vi "Create All Message Queues.vi"(8 "error in (no error)":errorcluster, 11 "Process Name":string) -> (0 "error out":errorcluster, 3 "Message Queues":T1)   [LabVIEW 2018, in "4-20mA Module.lvlib"]
uses:
  4-20mA Module.lvlib
  Controls/4-20mA Message Queues.ctl
  support/Message Queue/Message Cluster.ctl
  Config Module/Controls/OP Window Display.ctl
  Controls/4-20mA Display Cluster.ctl
  support/Message Queue/Enqueue Message (Single).vi
  support/Message Queue/Message Queue.lvlib
  Feed Module/Feed Module.lvlib
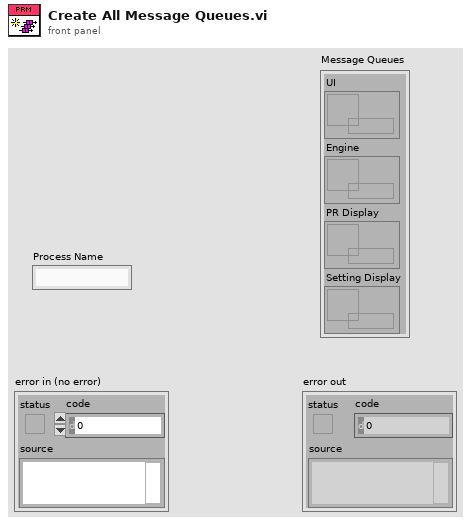
[diagram p1: front panel]
types:
  T1 = typedef "4-20mA Module.lvlib/4-20mA Message Queues.ctl" = cluster{"UI":refnum<queue>, "Engine":refnum<queue>, "PR Display":refnum<queue>, "Setting Display":refnum<queue>}
  T2 = typedef "4-20mA Module.lvlib/4-20mA Display Cluster.ctl" = cluster{"Input 4-20":dbl, "Output 4-20":dbl, "Cycle Period":dbl, "Status":enum16{"Off", "On", "Not Initialized"}}
  T3 = typedef "Feed Module.lvlib/OP Window Display.ctl" = cluster{"Flow":dbl, "Manual":dbl, "Pump Status":u16}
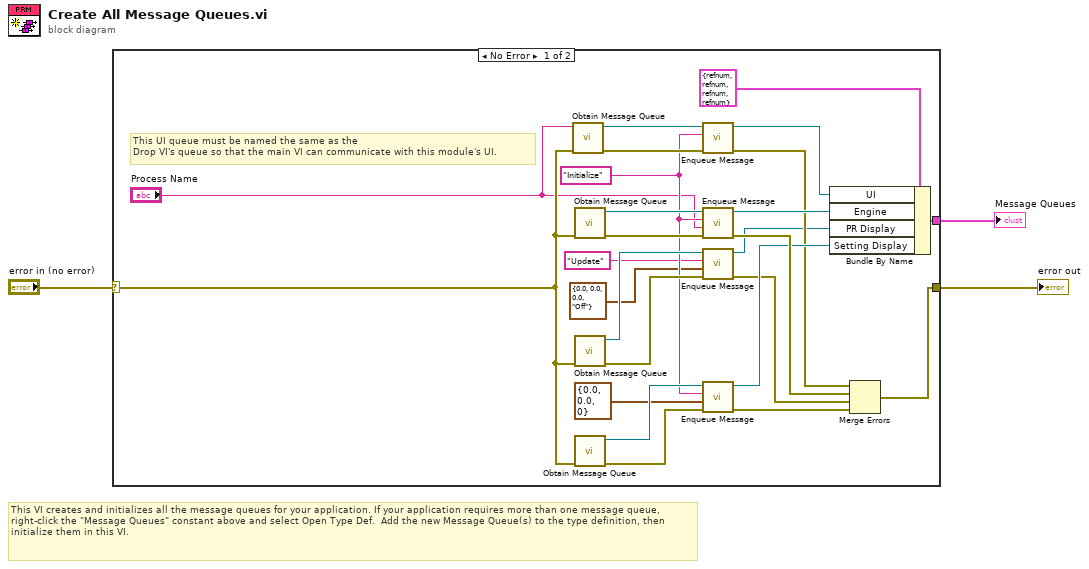
[diagram p0: block diagram]
diagram:
  # "This VI creates and initializes all the message queues for your application. If your application requires more than one message queue, right-click the \"Message Queues\" constant above and select Open Type Def.  Add the new Message Queue(s) to the type definition, then initialize them in this VI."
  n1 = case shown="No Error" "error in (no error)" {
    selector: "error in (no error)" -> [w14 w29]
    tunnel: [w25 w29] -> w3
    tunnel: [w28 _] -> w2
    frame No Error {
      w11 = "Initialize" ("Message")
      # "This UI queue must be named the same as the \nDrop VI's queue so that the main VI can communicate with this module's UI."
      n2 = call "Obtain Message Queue.vi"("error in (no error)"=w14, "name (unnamed)"="Process Name") -> ("error out"=w27:errorcluster, "Message Queue"=w26:refnum<queue>)  [unwired: 8 in]
      n3 = call "Obtain Message Queue.vi"("error in (no error)"=w14) -> ("error out"=w23:errorcluster, "Message Queue"=w24:refnum<queue>)  [unwired: 9 in]
      n4 = call "Obtain Message Queue.vi"("error in (no error)"=w14) -> ("error out"=w20:errorcluster, "Message Queue"=w19:refnum<queue>)  [unwired: 9 in]
      n5 = call "Obtain Message Queue.vi"("error in (no error)"=w14) -> ("error out"=w18:errorcluster, "Message Queue"=w17:refnum<queue>)  [unwired: 9 in]
      n6 = call-poly "Enqueue Message.vi"("error in (no error)"=w27, "Message"=w11, "Message Queue"=w26) -> ("error out"=w8:errorcluster, "dup Message Queue"=w9:refnum<queue>)  [unwired: 7 in]
      n7 = call-poly "Enqueue Message.vi"("error in (no error)"=w23, "Message Data"="Process Name", "Message"=w11, "Message Queue"=w24) -> ("error out"=w21:errorcluster, "dup Message Queue"=w22:refnum<queue>)  [unwired: 6 in]
      n8 = call-poly "Enqueue Message.vi"("error in (no error)"=w20, "Message Data"=T2 {"Input 4-20"=0.0, "Output 4-20"=0.0, "Cycle Period"=0.0, "Status"=enum."Off"} ("PRM Display Cluster"), "Message"="Update", "Message Queue"=w19) -> ("error out"=w5:errorcluster, "dup Message Queue"=w6:refnum<queue>)  [unwired: 6 in]
      n9 = call-poly "Enqueue Message.vi"("error in (no error)"=w18, "Message Data"=T3 {"Flow"=0.0, "Manual"=0.0, "Pump Status"=0}, "Message"=w11, "Message Queue"=w17) -> ("error out"=w12:errorcluster, "dup Message Queue"=w15:refnum<queue>)  [unwired: 6 in]
      n10 = Bundle By Name(cluster=T1 {"UI"=refnum, "Engine"=refnum, "PR Display"=refnum, "Setting Display"=refnum} ("Message Queues"), "UI"=w9, "Engine"=w22, "PR Display"=w6, "Setting Display"=w15) -> (w28:T1)
      n11 = Merge Errors(w8, w21, w5, w12) -> (w25:errorcluster)
    }
    frame Error {
    }
  }
  "Message Queues" <- w2
  "error out" <- w3
